vi "configure.vi"(8 "error in (no error)":errorcluster, 9 "Value":i32, 10 "ILC":refnum<class "ILC.lvclass">, 11 "ConfigureILCGPIStrategy in":refnum<class "ConfigureILCGPIStrategy.lvclass">) -> (0 "error out":errorcluster, 3 "ConfigureILCGPIStrategy out":refnum<class "ConfigureILCGPIStrategy.lvclass">)   [LabVIEW 2015, in "ConfigureILCGPIStrategy.lvclass"]
uses:
  ConfigureILCGPIStrategy.lvclass
  <userlib>/Common/ILC/ILC/ILC.lvclass
  ConfigureILCGPIStrategy.lvclass/ConfigureILCGPIStrategy.ctl
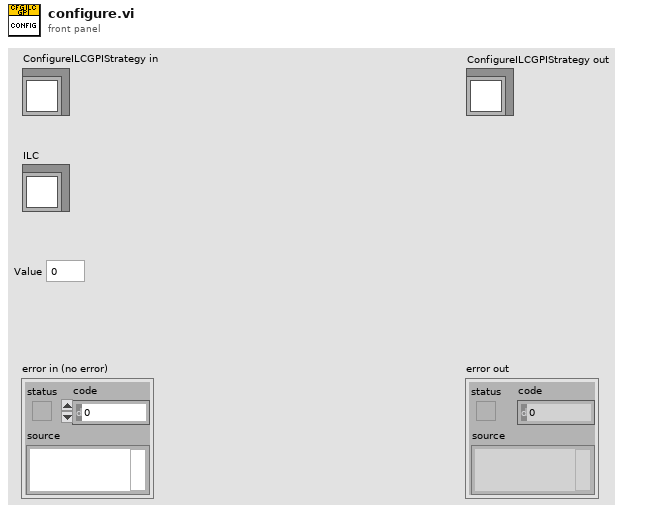
[diagram p1: front panel]
types:
  T1 = typedef "ILCBTTypedefs.lvlib/MUX Signals.ctl" = cluster{"MUX_A0 DAQ Channel to Write":refnum<k21>, "MUX_A1 DAQ Channel to Write":refnum<k21>}
  T2 = typedef "ILCBTTypedefs.lvlib/MUX Settings.ctl" = cluster{"MUX_AO":T3, "MUX_A1":T3}
  T3 = typedef "ILCBTTypedefs.lvlib/Digital Signal Level.ctl" = enum16{"Low", "High"}
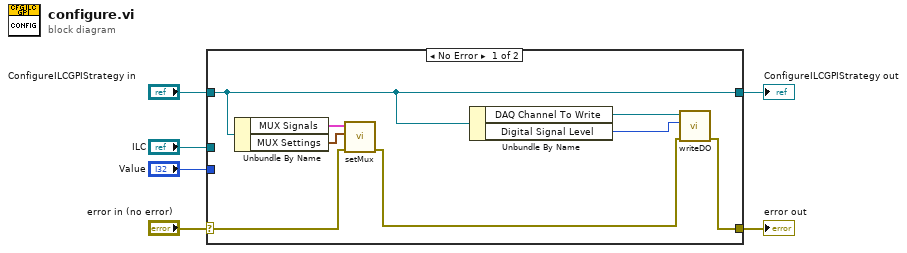
[diagram p0: block diagram]
diagram:
  n1 = case shown="No Error" "error in (no error)" {
    selector: "error in (no error)" -> [w13 w16]
    tunnel: [w8 w16] -> w5
    tunnel: [w11 w15] -> w3
    tunnel: "ConfigureILCGPIStrategy in" -> [w11 w15]
    tunnel: "ILC" -> [_ _]
    tunnel: "Value" -> [_ _]
    frame No Error {
      n2 = Unbundle By Name(w11) -> ("MUX Signals"=w14:T1, "MUX Settings"=w7:T2)
      n3 = call "setMux.vi"("error in (no error)"=w13, "MUX Settings"=w7, "MUX Signals"=w14) -> ("error out"=w9:errorcluster)  [unwired: 8 in]
      n4 = Unbundle By Name(w11) -> ("DAQ Channel To Write"=w10:refnum<k21>, "Digital Signal Level"=w12:T3)
      n5 = call "writeDO.vi"("error in"=w9, "Digital Signal Level"=w12, "DAQmx Global Channel"=w10) -> ("error out"=w8:errorcluster)  [unwired: 8 in]
    }
    frame Error {
    }
  }
  "error out" <- w5
  "ConfigureILCGPIStrategy out" <- w3
